vi "zad1.vi"() -> ()   [LabVIEW 2018]
doc: "Use this template to build a producer/consumer design pattern with events to produce queue items. Use this design pattern instead of the User Interface Event Handler pattern for user interfaces when you want to execute code asynchronously in response to an event without slowing the user interface responsiveness."
uses:
  <vilib>/Analysis/NI_AALBase.lvlib
panel:
  out "Waveform Chart":dbl[](graph)
  in  "Cluster":T1={"amplituda"=10, "czestotliwosc"=27, "Offset"=5, "sygnal - rodzaj"=enum."Sinus"}
  in  "Generate sinus":bool
  in  "stop":bool
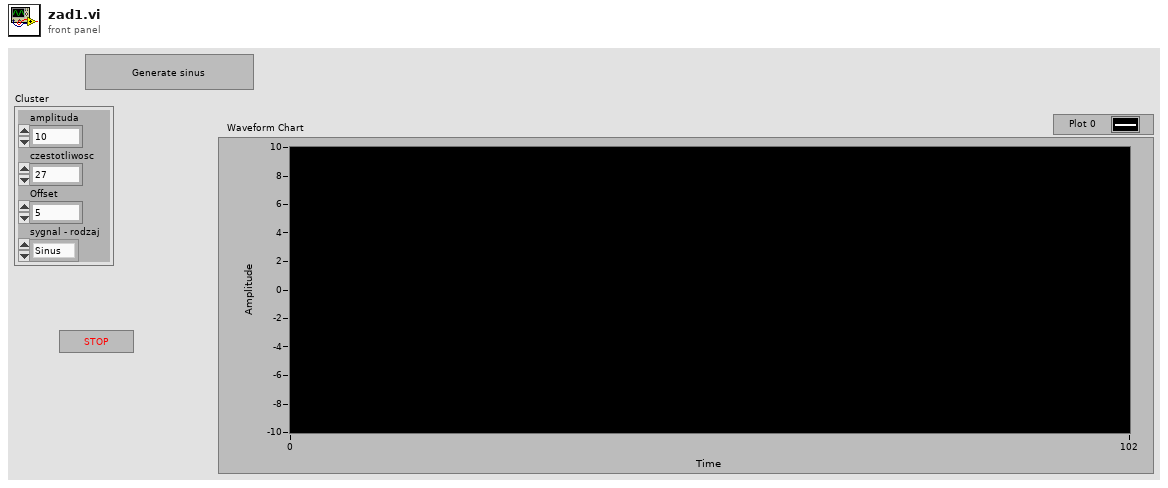
[diagram p1: front panel]
types:
  T1 = cluster{"amplituda":i32, "czestotliwosc":i32, "Offset":i32, "sygnal - rodzaj":enum16{"Sinus", "Kwadratowy"}}
  T2 = cluster{"Amplituda":i32, "Czesotliwosc":i32, "Offset":i32, "sygnal - rodzaj":enum16{"Sinus", "Kwadratowy"}}
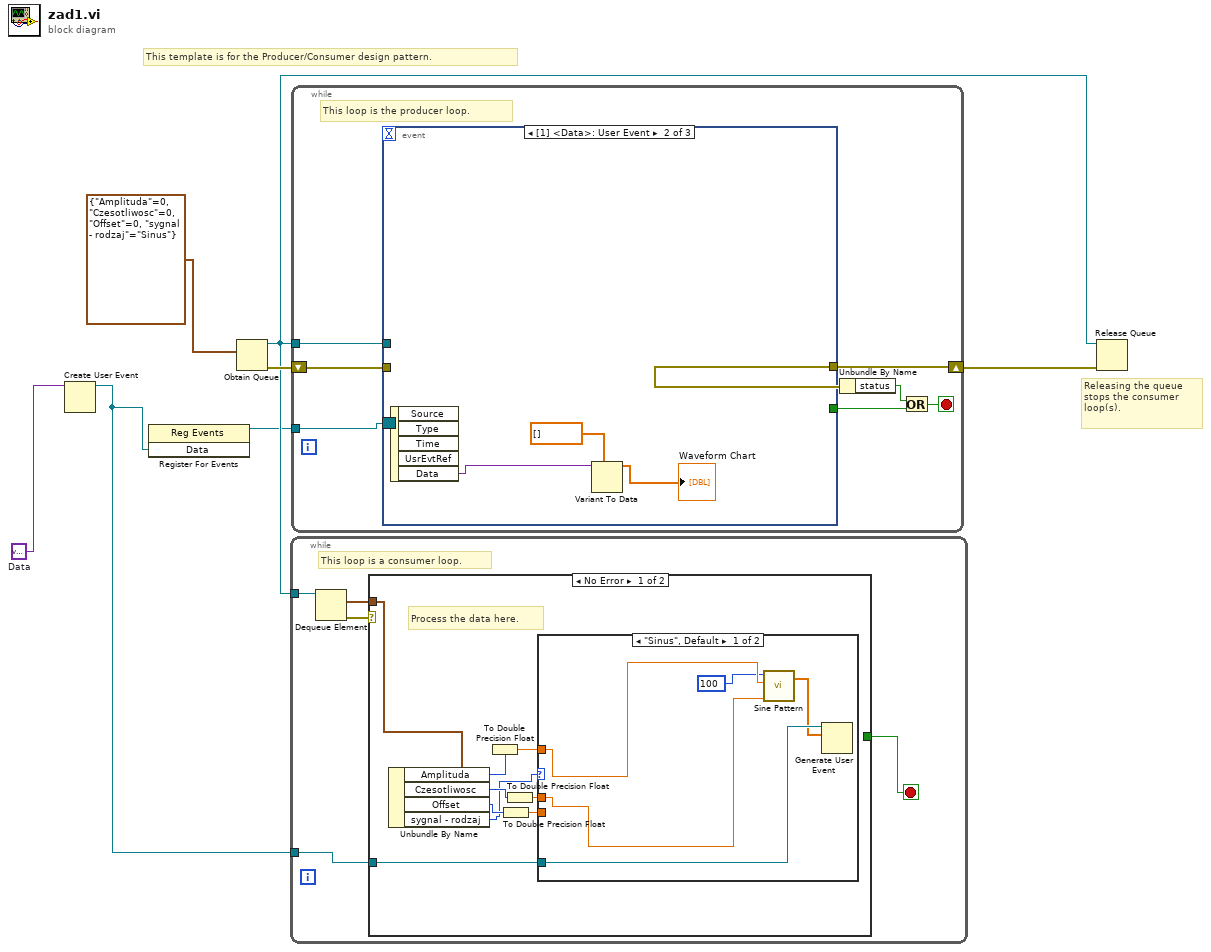
[diagram p0: block diagram]
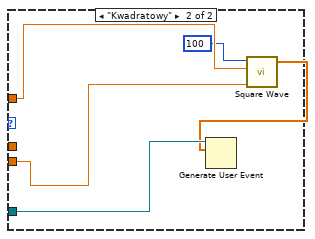
[diagram p2: hidden frame]
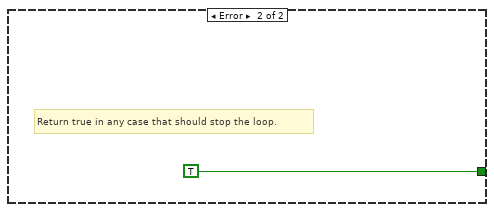
[diagram p3: hidden frame]
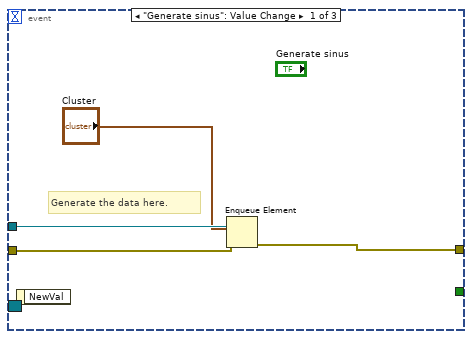
[diagram p4: hidden frame]
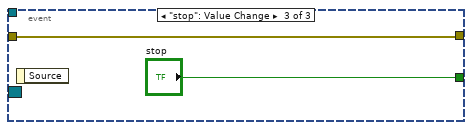
[diagram p5: hidden frame]
diagram:
  w3 = variant  # Data
  # "Releasing the queue stops the consumer loop(s)."
  # "This template is for the Producer/Consumer design pattern."
  n1 = Create User Event(user event datatype=w3) -> (user event=w2:refnum<user-event>)  [unwired: 1 in, 1 out]
  n2 = register-events(w2) -> (reference out=w1:refnum<event-registration>)  [unwired: 2 in, 1 out]
  n3 = Obtain Queue(element data type=T2 {"Amplituda"=0, "Czesotliwosc"=0, "Offset"=0, "sygnal - rodzaj"=enum."Sinus"}) -> (queue out=w5:refnum<queue>, error out=w7:errorcluster)  [unwired: 4 in, 1 out]
  n4 = while {
    tunnel: w5 -> [w12]
    tunnel: w2 -> [w8]
    stop <- w9 stop-if-true
    # "This loop is a consumer loop."
    n5 = Dequeue Element(queue=w12) -> (element=w10:T2, error out=w11:errorcluster)  [unwired: 2 in, 2 out]
    n6 = case shown="No Error" w11 {
      tunnel: w10 -> [w21 _]
      tunnel: [_ TRUE] -> w9
      tunnel: w8 -> [w13 _]
      frame No Error {
        # "Process the data here."
        n7 = Unbundle By Name(w21) -> ("Amplituda"=w19:i32, "Czesotliwosc"=w20:i32, "Offset"=w18:i32, "sygnal - rodzaj"=w15:enum16{"Sinus", "Kwadratowy"})
        n8 = To Double Precision Float(number=w19) -> (double precision float=w14:dbl)
        n9 = To Double Precision Float(number=w18) -> (double precision float=w16:dbl)
        n10 = To Double Precision Float(number=w20) -> (double precision float=w17:dbl)
        n11 = case shown="\"Sinus\", Default" w15 {
          tunnel: w17 -> [w25 _]
          tunnel: w16 -> [_ w28]
          tunnel: w14 -> [w24 w30]
          tunnel: w13 -> [w26 w31]
          frame "Sinus", Default {
            n12 = call <vilib>:"Sine Pattern.vi"("cycles"=w25, "amplitude"=w24, "samples"=100) -> ("Sinusoidal Pattern"=w23:dbl[])  [unwired: 1 in, 1 out]
            n13 = Generate User Event(user event=w26, event data cluster=w23) -> ()  [unwired: 2 in, 2 out]
          }
          frame "Kwadratowy" {
            n14 = call <vilib>:"Square Wave.vi"("samples"=100, "amplitude"=w30, "phase in"=w28) -> ("square wave"=w29:dbl[])  [unwired: 3 in, 2 out]
            n15 = Generate User Event(user event=w31, event data cluster=w29) -> ()  [unwired: 2 in, 2 out]
          }
        }
      }
      frame Error {
        # "Return true in any case that should stop the loop."
      }
    }
  }
  n16 = while {
    shift-right: [w35] -> w6
    shift-left: w7 -> [w38]
    tunnel: w5 -> [w39]
    tunnel: w1 -> [w33]
    stop <- w36 stop-if-true
    # "This loop is the producer loop."
    n17 = event shown="[1] <Data>: User Event" {
      selector: w33 -> [_ _ _]
      dyn-events: _ -> [_ _ _]
      timeout: _ -> [_ _ _]
      tunnel: w39 -> [w43 _ _]
      tunnel: w38 -> [w42 _ w47]
      tunnel: [w41 _ w47] -> w35
      tunnel: [_ _ "stop"] -> w37
      event "Generate sinus": Value Change {
        # "Generate the data here."
        n18 = event-data() -> ()  [unwired: 1 in, 1 out]
        n19 = Enqueue Element(queue=w43, element="Cluster", error in (no error)=w42) -> (error out=w41:errorcluster)  [unwired: 1 in, 2 out]
      }
      event User Event {
        n20 = event-data() -> ("Data"=w46:variant)  [unwired: 1 in, 4 out]
        n21 = Variant To Data(type=dbl[] [], Variant=w46) -> (data=→"Waveform Chart":dbl[])  [unwired: 1 in, 1 out]
      }
      event "stop": Value Change {
        n22 = event-data() -> ()  [unwired: 1 in, 1 out]
      }
    }
    n23 = Unbundle By Name(w35) -> ("status"=w34:bool)
    n24 = Or(x=w34, y=w37) -> (x .or. y?=w36:bool)
  }
  n25 = Release Queue(queue=w5, error in (no error)=w6) -> ()  [unwired: 1 in, 3 out]
